vi "dfd_DFXPSimu Add (ss).vi"(7 "op params":T1={"source"=0, "is floating?"=FALSE, "o-mode"=enum."Wrap", "q-mode"=enum."Truncation", "wl"=1, "high limit"=0, "low limit"=0, "iwl"=0, "sign?"=TRUE} {"source" items=["Coef a/k"=0, "Coef b/v"=7, "Input"=1, "Output"=2, "Multiplicand"=3, "Product"=4, "Sum"=5, "Delay"=6, "Gain"=8]}, 8 "filtering statistics in":T5(array[cluster]) {"statistics information"."min value" format="%.2f"; "statistics information"."max value" format="%.2f"; "Quantizer Source" items=["Coefficients a/k"=0, "Coefficients b/v"=7, "Input"=1, "Output"=2, "Multiplicand"=3, "Product"=4, "Sum"=5, "Delay"=6]}, 10 "value in 2":T6={"value"=0, "wl"=0, "iwl"=0, "Signed"=TRUE} {"value" format="%.0x"}, 11 "value in 1":T6={"value"=0, "wl"=0, "iwl"=0, "Signed"=TRUE} {"value" format="%.0x"}) -> (0 "filtering statistics out":T5(array[cluster]) {"statistics information"."min value" format="%.2f"; "statistics information"."max value" format="%.2f"; "Quantizer Source" items=["Coefficients a/k"=0, "Coefficients b/v"=7, "Input"=1, "Output"=2, "Multiplicand"=3, "Product"=4, "Sum"=5, "Delay"=6]}, 3 "value out":T6={"value"=0, "wl"=0, "iwl"=0, "Signed"=TRUE} {"value" format="%.0x"})   [LabVIEW 2017, in "NI_DigFilter_FXP.lvlib"]
uses:
  <vilib>/addons/Digital Filter Design/NI_DigFilter_FXP.lvlib
  <vilib>/addons/Digital Filter Design/_Objects.llb/dfd_DFXP Data Type (scaler).ctl
  <vilib>/addons/Digital Filter Design/_Objects.llb/DFD Quantization Sources.ctl
  <vilib>/addons/Digital Filter Design/_Objects.llb/DFD FXP Statistics Data.ctl
  <vilib>/addons/Digital Filter Design/_Objects.llb/dfd_DFXP Operation Parameter.ctl
  <vilib>/addons/Digital Filter Design/_Objects.llb/dfd_Internal Quantization Srcs.ctl
  <vilib>/addons/Digital Filter Design/NI_DigFilterLicensed.lvlib
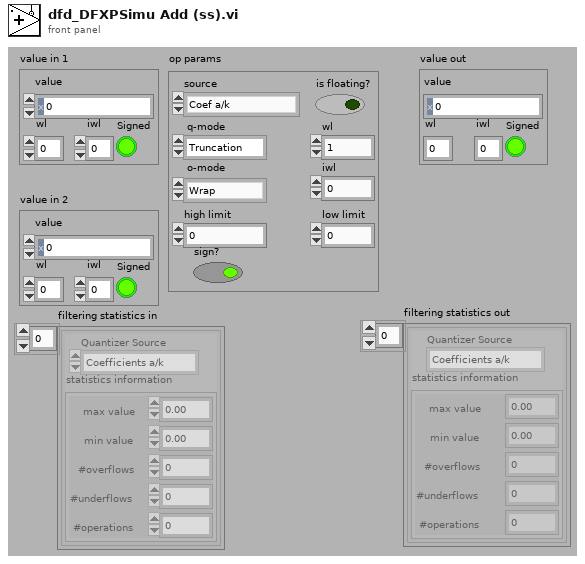
[diagram p1: front panel]
types:
  T1 = typedef "dfd_DFXP Operation Parameter.ctl" = cluster{"source":T2, "is floating?":bool, "o-mode":enum16{"Saturation", "Wrap"}, "q-mode":enum16{"Nearest", "Truncation"}, "wl":i16, "high limit":i64, "low limit":i64, "iwl":i16, "sign?":bool}
  T2 = typedef "NI_DigFilterLicensed.lvlib/dfd_Internal Quantization Srcs.ctl" = u16
  T3 = typedef "NI_DigFilterLicensed.lvlib/DFD Quantization Sources.ctl" = u16
  T4 = typedef "NI_DigFilterLicensed.lvlib/DFD FXP Statistics Data.ctl" = cluster{"max value":ext, "min value":ext, "#overflows":i32, "#underflows":i32, "#operations":i32}
  T5 = cluster{"Quantizer Source":T3, "statistics information":T4}[]
  T6 = typedef "dfd_DFXP Data Type (scaler).ctl" = cluster{"value":i64, "wl":i16, "iwl":i16, "Signed":bool}
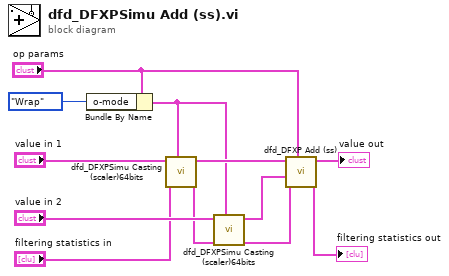
[diagram p0: block diagram]
diagram:
  n1 = Bundle By Name(cluster="op params", "o-mode"=enum16{"Saturation", "Wrap"}."Wrap" ("o_mode")) -> (w2:T1)
  n2 = call <vilib>:"dfd_DFXPSimu Casting (scaler)64bits.vi"("op params"=w2, "filtering statistics in"="filtering statistics in", "Value in"="value in 1") -> ("filtering statistics out"=w6:T5, "Value out"=w4:T6)  [unwired: 1 in, 6 out]
  n3 = call <vilib>:"dfd_DFXPSimu Casting (scaler)64bits.vi"("op params"=w2, "filtering statistics in"=w6, "Value in"="value in 2") -> ("filtering statistics out"=w5:T5, "Value out"=w3:T6)  [unwired: 1 in, 6 out]
  n4 = call <vilib>:"dfd_DFXP Add (ss).vi"("op params"="op params", "filtering statistics in"=w5, "Value in 2"=w3, "Value in"=w4) -> ("filtering statistics out"=→"filtering statistics out":T5, "Value out"=→"value out":T6)  [unwired: 1 in, 5 out]
